vi "PS4ControlReal.vi"(7 "Forward Speed Limit [rad/s] (10.7 r/s)":dbl=10.7 format="%#_13g", 8 "Error In":errorcluster, 11 "PS4 Controller Ref In":T1) -> (0 "Error Out":errorcluster, 1 "right motor out":dbl, 2 "left motor out":dbl, 3 "PS4 Controller Ref Out":T1)   [LabVIEW 2012]
uses:
  <vilib>/MakerHub/PS4-Controller/Private/Type Defs/PS4 Controller Ref.ctl
  <vilib>/MakerHub/PS4-Controller/LMH-PS4.lvlib
panel:
  # "Max. 15.7 [rad/s]"
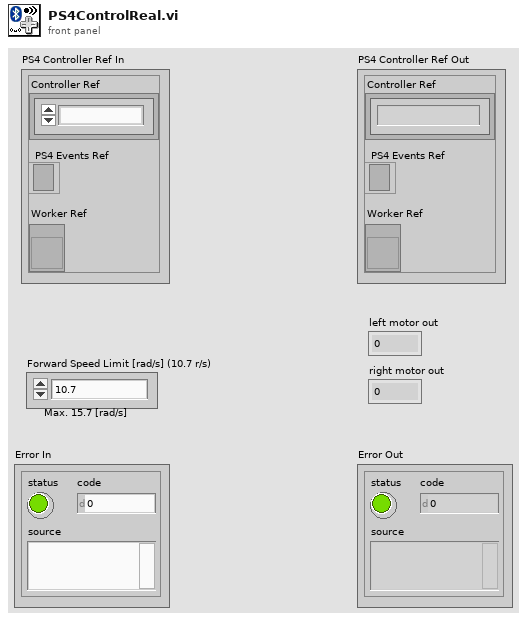
[diagram p1: front panel]
types:
  T1 = typedef "LMH-PS4.lvlib/PS4 Controller Ref.ctl" = cluster{"Controller Ref":refnum<k1>, "PS4 Events Ref":refnum<event-registration>, "Worker Ref":refnum<vi>}
  T2 = typedef "LMH-PS4.lvlib/Axis.ctl" = cluster{"Left Thumbstick":cluster{"X Axis":i32, "Y Axis":i32}, "Right Thumbstick":cluster{"X Axis":i32, "Y Axis":i32}, "L2":i32, "R2":i32, "D-Pad":T3}
  T3 = typedef "LMH-PS4.lvlib/DPad Enum.ctl" = enum16{"Idle", "Up", "Up / Right", "Right", "Down / Right", "Down", "Down / Left", "Left", "Up / Left"}
  T4 = typedef "LMH-PS4.lvlib/Buttons.ctl" = cluster{"Square":bool, "X":bool, "Circle":bool, "Triangle":bool, "L1":bool, "R1":bool, "L2":bool, "R2":bool, "Share":bool, "Options":bool, "Left Thumbstick":bool, "Right Thumbstick":bool, "Playstation Button":bool, "Pad":bool}
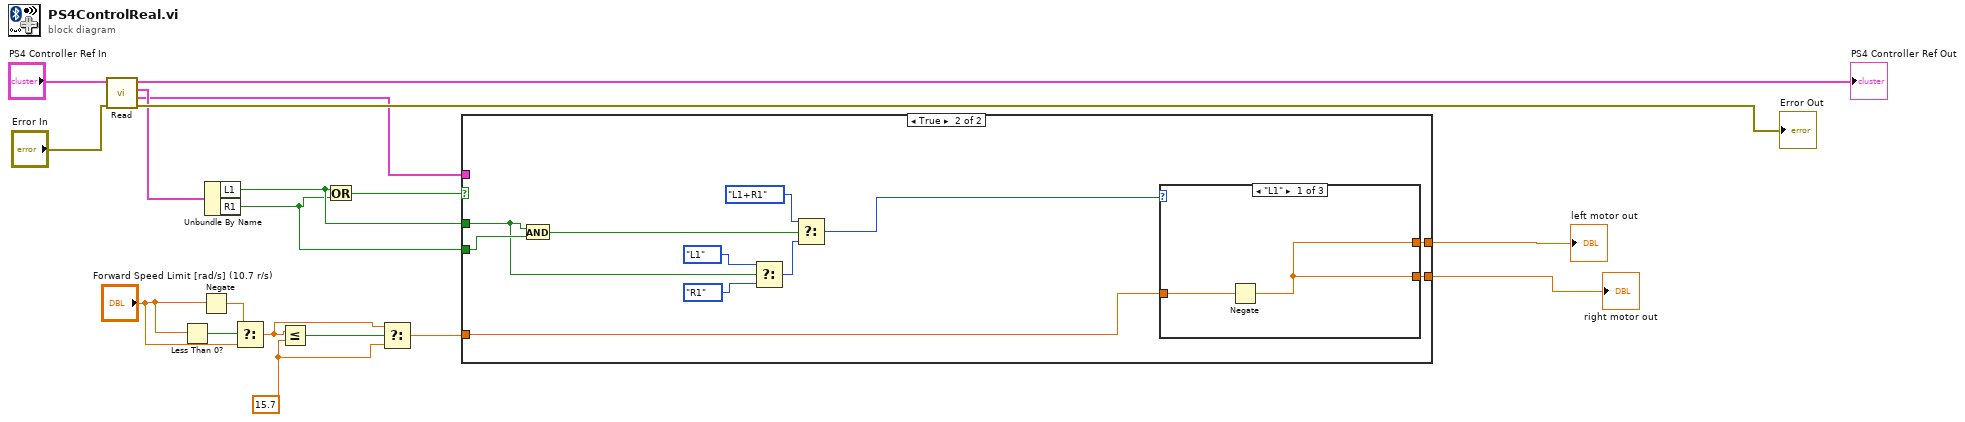
[diagram p0: block diagram]
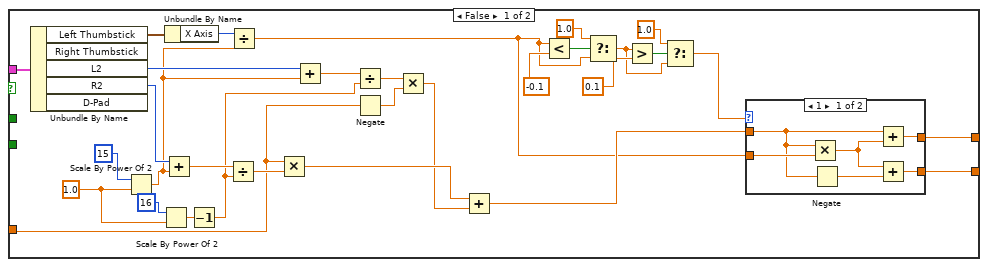
[diagram p2: hidden frame]
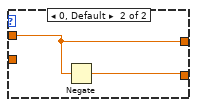
[diagram p3: hidden frame]
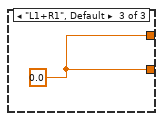
[diagram p5: hidden frame]
diagram:
  w2 = 15.7 ("y")
  n1 = call <vilib>:"Read.vi"("Error In"="Error In", "PS4 Controller Ref"="PS4 Controller Ref In") -> ("Error Out"=→"Error Out":errorcluster, "All Axis"=w15:T2, "Buttons"=w16:T4, "PS4 Controller Ref"=→"PS4 Controller Ref Out":T1)  [unwired: 6 in]
  n2 = Less Than 0?(x="Forward Speed Limit [rad/s] (10.7 r/s)") -> (x < 0?=w7:bool)
  n3 = Negate(x="Forward Speed Limit [rad/s] (10.7 r/s)") -> (-x=w6:dbl)
  n4 = Unbundle By Name(w16) -> ("L1"=w13:bool, "R1"=w12:bool)
  n5 = Select(t=w6, s=w7, f="Forward Speed Limit [rad/s] (10.7 r/s)") -> (s? t:f=w3:dbl)
  n6 = Less Or Equal?(x=w3, y=w2) -> (x <= y?=w4:bool)
  n7 = Or(x=w13, y=w12) -> (x .or. y?=w14:bool)
  n8 = Select(t=w3, s=w4, f=w2) -> (s? t:f=w1:dbl)
  n9 = case shown="True" w14 {
    tunnel: w15 -> [w49 _]
    tunnel: w13 -> [_ w63]
    tunnel: w12 -> [_ w68]
    tunnel: [w27 w60] -> w9
    tunnel: [w26 w59] -> w10
    tunnel: w1 -> [w19 w58]
    frame False {
      w23 = 1.0
      n10 = Unbundle By Name(w49) -> ("Left Thumbstick"=w43:cluster{"X Axis":i32, "Y Axis":i32}, "L2"=w48:i32, "R2"=w45:i32)  [unwired: 2 out]
      n11 = Scale By Power Of 2(n=i16 15, x=w23) -> (x*2^n=w24:dbl)
      n12 = Scale By Power Of 2(n=i16 16, x=w23) -> (x*2^n=w21:dbl)
      n13 = Add(x=w45, y=w24) -> (x+y=w46:dbl)
      n14 = Unbundle By Name(w43) -> ("X Axis"=w42:i32)
      n15 = Decrement(x=w21) -> (x-1=w20:dbl)
      n16 = Divide(x=w46, y=w20) -> (x/y=w28:dbl)
      n17 = Divide(x=w42, y=w24) -> (x/y=w32:dbl)
      n18 = Multiply(x=w19, y=w28) -> (x*y=w31:dbl)
      n19 = Add(x=w48, y=w24) -> (x+y=w47:dbl)
      n20 = Divide(x=w47, y=w20) -> (x/y=w44:dbl)
      n21 = Negate(x=w19) -> (-x=w29:dbl)
      n22 = Multiply(x=w44, y=w29) -> (x*y=w30:dbl)
      n23 = Add(x=w31, y=w30) -> (x+y=w39:dbl)
      n24 = Less?(x=w32, y=-0.1) -> (x < y?=w41:bool)
      n25 = Select(t=1.0, s=w41, f=w32) -> (s? t:f=w34:dbl)
      n26 = Greater?(x=w34, y=0.1) -> (0:w37:bool)
      n27 = Select(t=1.0, s=w37, f=w34) -> (s? t:f=w33:dbl)
      n28 = case shown="1" w33 {
        tunnel: w39 -> [w54 w57]
        tunnel: w32 -> [w55 _]
        tunnel: [w51 w57] -> w27
        tunnel: [w50 w56] -> w26
        frame 1 {
          n29 = Multiply(x=w54, y=w55) -> (x*y=w53:dbl)
          n30 = Negate(x=w54) -> (-x=w52:dbl)
          n31 = Add(x=w54, y=w53) -> (x+y=w51:dbl)
          n32 = Add(x=w53, y=w52) -> (x+y=w50:dbl)
        }
        frame 0, Default {
          n33 = Negate(x=w57) -> (-x=w56:dbl)
        }
      }
    }
    frame True {
      n34 = And(x=w63, y=w68) -> (x .and. y?=w67:bool)
      n35 = Select(t=enum16{"L1", "R1", "L1+R1"}."L1", s=w63, f=enum16{"L1", "R1", "L1+R1"}."R1") -> (s? t:f=w64:enum16{"L1", "R1", "L1+R1"})
      n36 = Select(t=enum16{"L1", "R1", "L1+R1"}."L1+R1", s=w67, f=w64) -> (s? t:f=w65:enum16{"L1", "R1", "L1+R1"})
      n37 = case shown="\"L1\"" w65 {
        tunnel: [w70 w71 w72] -> w59
        tunnel: [w70 w71 w72] -> w60
        tunnel: w58 -> [w69 w71 _]
        frame "L1" {
          n38 = Negate(x=w69) -> (-x=w70:dbl)
        }
        frame "R1" {
        }
        frame "L1+R1", Default {
          w72 = 0.0 ("left motor ccw velocity (rad/s)")
        }
      }
    }
  }
  "right motor out" <- w10
  "left motor out" <- w9
